vi "createBackup.vi"(0 "reference in":refnum<class "excelFile.lvclass">, 5 "error in (no error)":errorcluster) -> (14 "reference out":refnum<class "excelFile.lvclass">, 19 "error out":errorcluster)   [LabVIEW 2016, in "excelFile.lvclass"]
uses:
  excelFile.lvclass
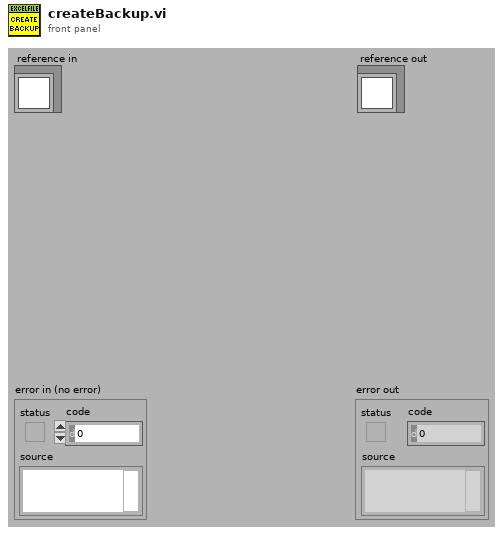
[diagram p1: front panel]
types:
  T1 = typedef "excelFile.lvclass/ObjectAttributesRef.ctl" = refnum<data-value>
  T2 = typedef "excelFile.lvclass/ObjectAttributes.ctl" = cluster{"MyAttribute":dbl, "path":string, "Refnum Excel":cluster{"Excel._Application":refnum<k7>, "Workbooks":refnum<k7>, "Open":refnum<k7>}, "data":string[][][], "save":bool, "fileType":T3, "rowsColor":u32[], "python_ref":refnum<class "python.lvclass">, "items_rows":i32[], "excel_range":i32[][], "TSR":cluster{"number":string, "TSR_path":path, "service_path":path, "email_to":string}, "excel_already_opened?":bool, "file_already_opened?":bool, "excel_protected_opened?":bool}
  T3 = typedef "excelFile.lvclass/fileType.ctl" = enum16{"devices", "items", "partsTracking", "TSR"}
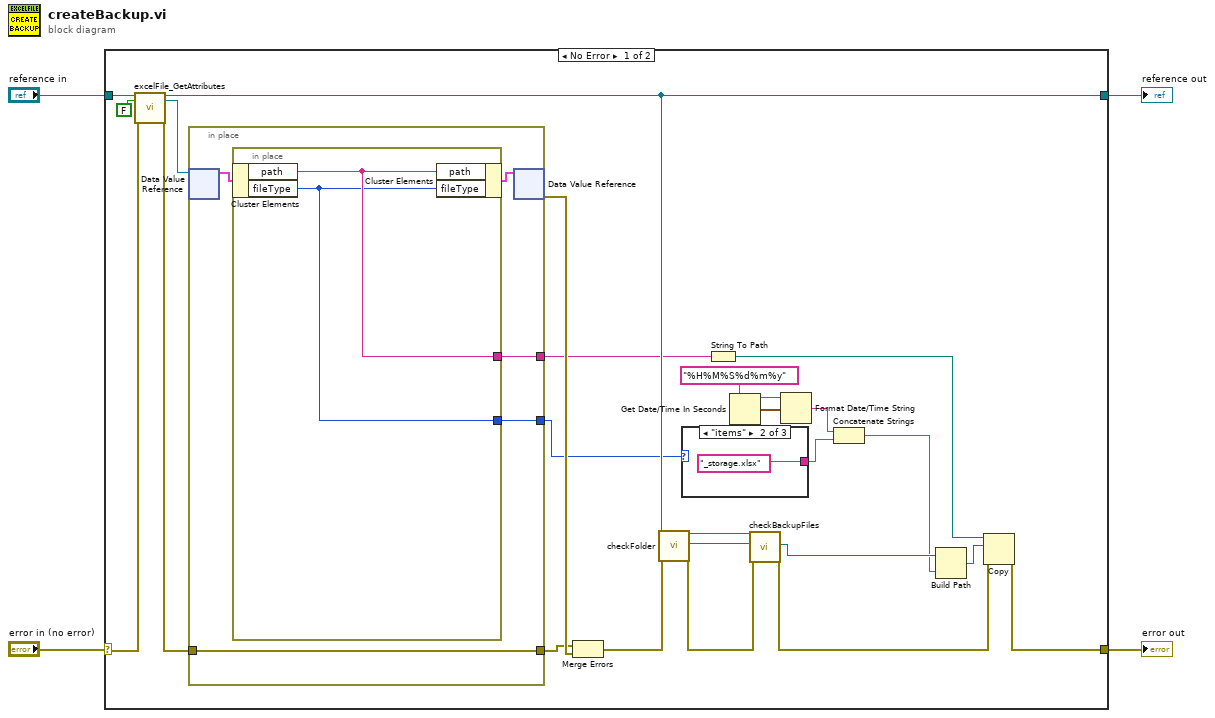
[diagram p0: block diagram]
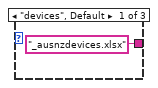
[diagram p2: hidden frame]
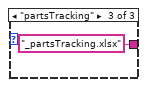
[diagram p3: hidden frame]
diagram:
  n1 = case shown="No Error" "error in (no error)" {
    selector: "error in (no error)" -> [w24 w40]
    tunnel: [w15 w40] -> w3
    tunnel: [w21 w39] -> w1
    tunnel: "reference in" -> [w26 w39]
    frame No Error {
      n2 = call "excelFile_GetAttributes.vi"("reference in"=w26, "return data? (T)"=FALSE, "error in (no error)"=w24) -> ("reference out"=w21:refnum<class "excelFile.lvclass">, "attributes ref"=w22:T1, "error out"=w23:errorcluster)  [unwired: 13 in, 1 out]
      n3 = in-place {
        in-place-border: w23 -> [w34]
        in-place-border: [w34] -> w27
        in-place-border: [w33] -> w14
        in-place-border: [w32] -> w8
        n4 = in-place-dvr #1(w22) -> (w35:T2)  [unwired: 1 out]
        n5 = in-place {
          in-place-border: [w38] -> w33
          in-place-border: [w37] -> w32
          n6 = in-place-cluster #2(w35) -> ("path"=w38:string, "fileType"=w37:T3)
          n7 = in-place-cluster #2("path"=w38, "fileType"=w37) -> (w36:T2)
        }
        n8 = in-place-dvr #1(w36) -> (w28:errorcluster)  [unwired: 1 out]
      }
      n9 = Merge Errors(w27, w28) -> (w20:errorcluster)
      n10 = call "checkFolder.vi"("reference in"=w21, "error in (no error)"=w20) -> ("reference out"=w19:refnum<class "excelFile.lvclass">, "backup_path"=w18:path, "error out"=w17:errorcluster)  [unwired: 15 in]
      n11 = case shown="\"items\"" w8 {
        tunnel: ["_ausnzdevices.xlsx" "_storage.xlsx" "_partsTracking.xlsx"] -> w6
        frame "devices", Default {
        }
        frame "items" {
        }
        frame "partsTracking" {
        }
      }
      n12 = String To Path(string=w14) -> (path=w13:path)
      n13 = Get Date/Time In Seconds() -> (seconds since 1Jan1904=w10:timestamp)
      n14 = call "checkBackupFiles.vi"("reference in"=w19, "backup_path"=w18, "error in (no error)"=w17) -> ("backup_path"=w11:path, "error out"=w16:errorcluster)  [unwired: 14 in, 1 out]
      n15 = Format Date/Time String(time format string (%c)="%H%M%S%d%m%y", seconds (now)=w10) -> (date/time string=w7:string)  [unwired: 1 in]
      n16 = Concatenate Strings(w7, w6) -> (w5:string)
      n17 = Build Path(base path=w11, name or relative path=w5) -> (appended path=w12:path)
      n18 = Copy(8:w16, 10:w12, 11:w13) -> (0:w15:errorcluster)  [unwired: 2 in, 2 out]
    }
    frame Error {
    }
  }
  "error out" <- w3
  "reference out" <- w1
